vi "Open Sensors.vi"   [LabVIEW 2014]
uses:
  Robot Global Data.vi
  <vilib>/Rock Robotics/WPI/Counter/WPI_CounterDigitalInputToDigitalSource.vi
  <vilib>/Rock Robotics/WPI/Switch/WPI_SwitchOpenLimit.vi
types:
  T1 = typedef "FPGA_DIOChannel.ctl" = enum8{"DIO 0", "DIO 1", "DIO 2", "DIO 3", "DIO 4", "DIO 5", "DIO 6", "DIO 7", "DIO 8", "DIO 9", "DIO MXP 0", "DIO MXP 1", "DIO MXP 2", "DIO MXP 3", "DIO MXP 4", "DIO MXP 5", "DIO MXP 6", "DIO MXP 7", "DIO MXP 8", "DIO MXP 9", "DIO MXP 10", "DIO MXP 11", "DIO MXP 12", "DIO MXP 13", "DIO MXP 14", "DIO MXP 15", "Invalid"}
  T2 = cluster{"Lift Motors":cluster{"Left Lift":dbl, "Right Lift":dbl}, "Sensors":cluster{"Limit Switches":cluster{"Bottom IR":T1, "Top IR":T1}, "Encoders":cluster{"Lift Encoder A Pin":T1, "Lift Encoder B Pin":T1}}, "Solenoids":cluster{"Left Clamp FWD":dbl, "Right Clamp FWD":dbl, "Brake":dbl, "Left Clamp BCK":dbl, "Right Clamp BCK":dbl, "Left Clamp PModule":dbl, "Right Clamp PModule":dbl, "Brake PModule":dbl}, "Drive Motors":cluster{"Rear Left Motor":dbl, "Rear Right Motor":dbl, "Front Left Motor":dbl, "Front Right Motor":dbl}}
  T3 = typedef "WPI_DigitalInputDevRef.ctl" = cluster{"DevStatus":errorcluster, "DIO Channel":T1, "Controller":T4}
  T4 = typedef "FPGA_TypedefDigitalModule.ctl" = enum16{"Controller 1"}
  T5 = typedef "WPI_SwitchDevRef.ctl" = cluster{"DevStatus":errorcluster, "DIO Channel":T1, "Controller":T4, "CntIndex":T6, "Normally Closed":bool}
  T6 = typedef "FPGA_CounterCtrSystemIndex.ctl" = enum8{"Ctr 0", "Ctr 1", "Ctr 2", "Ctr 3", "Ctr 4", "Ctr 5", "Ctr 6", "Ctr 7", "Invalid"}
  T7 = typedef "FPGA_CounterEncoderSourceConvertionLVSourceType.ctl" = cluster{"DevStatus":errorcluster, "AnalogTriggerMode?":bool, "DigitalMode":cluster{"Controller":T4, "DIO Channel":T8}, "AnalogTriggerMode":cluster{"AnalogTriggerIndex":T9, "OutputType":T10}}
  T8 = typedef "FPGA_DIODigitalSourceChannel.ctl" = enum8{"DIO 0", "DIO 1", "DIO 2", "DIO 3", "DIO 4", "DIO 5", "DIO 6", "DIO 7", "DIO 8", "DIO 9", "DIO MXP 0", "DIO MXP 1", "DIO MXP 2", "DIO MXP 3", "DIO MXP 4", "DIO MXP 5", "DIO MXP 6", "DIO MXP 7", "DIO MXP 8", "DIO MXP 9", "DIO MXP 10", "DIO MXP 11", "DIO MXP 12", "DIO MXP 13", "DIO MXP 14", "DIO MXP 15", "Disabled"}
  T9 = typedef "FPGA_AnalogTriggerIndex.ctl" = enum8{"Trig 0", "Trig 1", "Trig 2", "Trig 3", "Trig 4", "Trig 5", "Trig 6", "Trig 7", "Invalid"}
  T10 = typedef "FPGA_AnalogTriggerOutType.ctl" = enum16{"InWindow", "TriggerState", "Rising", "Falling"}
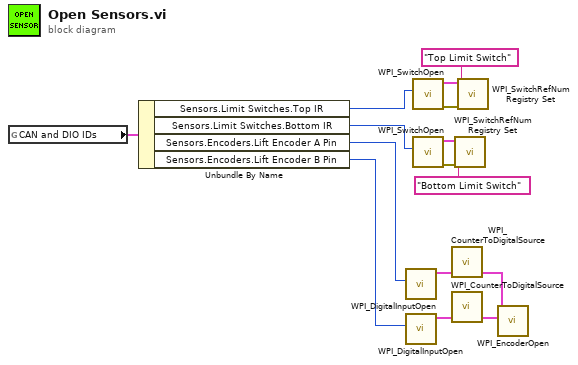
[diagram p0: block diagram]
diagram:
  n1 = global read "Robot Global Data.vi" "CAN and DIO IDs"() -> (w15:T2)
  n2 = Unbundle By Name(w15) -> ("Sensors.Limit Switches.Top IR"=w14:T1, "Sensors.Limit Switches.Bottom IR"=w13:T1, "Sensors.Encoders.Lift Encoder A Pin"=w2:T1, "Sensors.Encoders.Lift Encoder B Pin"=w1:T1)
  n3 = call <vilib>:"WPI_DigitalInputOpen.vi"("DIO Channel"=w2) -> ("DigitalInputDevRef"=w4:T3)  [unwired: 2 in, 8 out]
  n4 = call <vilib>:"WPI_DigitalInputOpen.vi"("DIO Channel"=w1) -> ("DigitalInputDevRef"=w5:T3)  [unwired: 2 in, 8 out]
  n5 = call-poly <vilib>:"WPI_SwitchOpen.vi"("DIO Channel"=w14) -> ("error out"=w12:errorcluster, "SwitchDevRef"=w11:T5)  [unwired: 9 in]
  n6 = call-poly <vilib>:"WPI_SwitchOpen.vi"("DIO Channel"=w13) -> ("error out"=w10:errorcluster, "SwitchDevRef"=w9:T5)  [unwired: 9 in]
  n7 = call-poly <vilib>:"WPI_CounterToDigitalSource.vi"("DigitalInputDevRef"=w4) -> ("Digital Source"=w3:T7)  [unwired: 6 out]
  n8 = call-poly <vilib>:"WPI_CounterToDigitalSource.vi"("DigitalInputDevRef"=w5) -> ("Digital Source"=w6:T7)  [unwired: 6 out]
  n9 = call <vilib>:"WPI_SwitchRefNum Registry Set.vi"("error in (no error)"=w10, "refnum name"="Bottom Limit Switch", "SwitchDevRef"=w9) -> ()  [unwired: 7 in, 2 out]
  n10 = call <vilib>:"WPI_SwitchRefNum Registry Set.vi"("error in (no error)"=w12, "refnum name"="Top Limit Switch", "SwitchDevRef"=w11) -> ()  [unwired: 7 in, 2 out]
  n11 = call <vilib>:"WPI_EncoderOpen.vi"("BSource"=w6, "ASource"=w3) -> ()  [unwired: 6 in, 4 out]
